vi "add_element(variant).vi"(8 "error in (no error)":errorcluster, 10 "element":cluster{"name":string, "address":string}, 11 "data store (variant)":variant) -> (0 "error out":errorcluster, 3 "data store (variant)":variant)   [LabVIEW 2016]
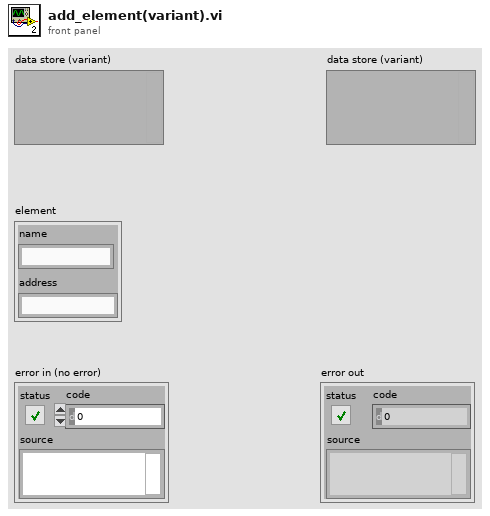
[diagram p1: front panel]
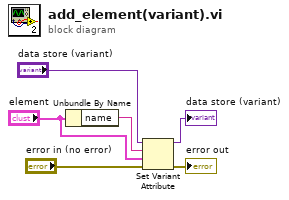
[diagram p0: block diagram]
diagram:
  n1 = Unbundle By Name("element") -> ("name"=w4:string)
  n2 = Set Variant Attribute(Variant="data store (variant)", name=w4, value="element", error in="error in (no error)") -> (Variant out=→"data store (variant)":variant, error out=→"error out":errorcluster)  [unwired: 1 out]
